vi "2016 Auto Drive Arm.vi"(0 "Left Side Speed":dbl, 2 "Right Side Speed":dbl, 3 "Arm Reference":T1, 5 "Arm Limits":T2, 6 "Left Side Reset":bool, 7 "Right Side Reset":bool, 8 "Left Upper Limit":dbl, 9 "Right Upper Limit":dbl, 10 "Left Lower Limit":dbl, 11 "Right Lower Limit":dbl) -> (14 "Encoder Status":T4, 16 "Encoder Status 2":T4, 19 "Arm Data":T3)   [LabVIEW 2015]
uses:
  <vilib>/Rock Robotics/WPI/Utilities/WPI_GetSetVariantRefNum.vi
  <vilib>/Rock Robotics/Network Tables/SD Write Numeric Array.vi
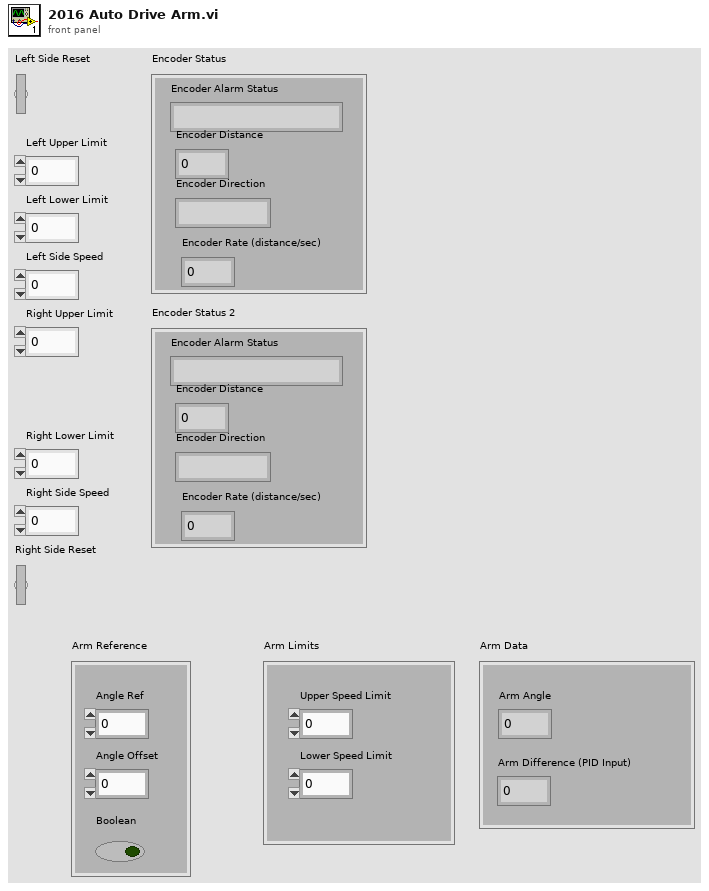
[diagram p1: front panel]
types:
  T1 = cluster{"Angle Ref":dbl, "Angle Offset":dbl, "Boolean":bool}
  T2 = cluster{"Upper Speed Limit":dbl, "Lower Speed Limit":dbl}
  T3 = cluster{"Arm Angle":dbl, "Arm Difference (PID Input)":dbl}
  T4 = cluster{"Encoder Alarm Status":string, "Encoder Distance":dbl, "Encoder Direction":string, "Encoder Rate (distance/sec)":dbl}
  T5 = typedef "WPI_PotentiometerDevRef.ctl" = cluster{"DevStatus":errorcluster, "Analog Channel":T6, "Invert Output":bool}
  T6 = typedef "FPGA_AIChannel.ctl" = enum8{"AI 0", "AI 1", "AI 2", "AI 3", "AI MXP 0", "AI MXP 1", "AI MXP 2", "AI MXP 3", "Invalid"}
  T7 = cluster{"P Gain":dbl, "I Gain":dbl, "D Gain":dbl, "t":dbl}
  T8 = cluster{"Arm Angle":dbl, "Angle Difference (PID Ref)":dbl}
  T9 = cluster{dbl, "Output offset":dbl, "Left Side Reset":bool}
  T10 = cluster{dbl, "Output offset":dbl, "Right Side Reset":bool}
  T11 = cluster{"Right Up Limit":dbl, "Right Lwr Limit":dbl}
  T12 = cluster{"Left Up Limit":dbl, "Left Lwr Limit":dbl}
  T13 = typedef "WPI_RobotDriveDevRef.ctl" = cluster{"DevStatus":errorcluster, "Motors[]":T14[], "Square Inputs":bool, "Max Output":dbl}
  T14 = typedef "WPI_MotorControlDeviceRef.ctl" = cluster{"DeviceStatus":errorcluster, "Type":T15, "PWM":cluster{"PWM Channel":T16, "DeadBand":T17}, "CAN":cluster{"Device Number":u8, "Control Mode":T18, "Semaphore":T19, "Max Vout":dbl, "TalonSRX Control Mode":T20}, "Invert":bool}
  T15 = typedef "WPI_MotorControlType.ctl" = enum16{"PWM", "CAN", "CANTalonSRX"}
  T16 = typedef "FPGA_DIOPWMChannel.ctl" = enum8{"PWM 0", "PWM 1", "PWM 2", "PWM 3", "PWM 4", "PWM 5", "PWM 6", "PWM 7", "PWM 8", "PWM 9", "PWM MXP 0", "PWM MXP 1", "PWM MXP 2", "PWM MXP 3", "PWM MXP 4", "PWM MXP 5", "PWM MXP 6", "PWM MXP 7", "PWM MXP 8", "PWM MXP 9", "Invalid"}
  T17 = typedef "WPI_PWMDeadband.ctl" = cluster{"Name":string, "maxPositivePwm":i32, "minPositivePwm":i32, "centerPwm":i32, "maxNegativePwm":i32, "minNegativePwm":i32, "angularRange":u16}
  T18 = typedef "WPI_CANJaguar_ControlMode.ctl" = enum8{"Percent VBus", "Current", "Speed", "Position", "Voltage"}
  T19 = typedef "Semaphore RefNum" = refnum<k1>
  T20 = typedef "WPI_CANTalonSRX_APIControlMode.ctl" = enum8{"Percent VBus", "Speed", "Position", "Slave", "Unchanged / Invalid", "Voltage Compensation", "Current", "Motion Profile"}
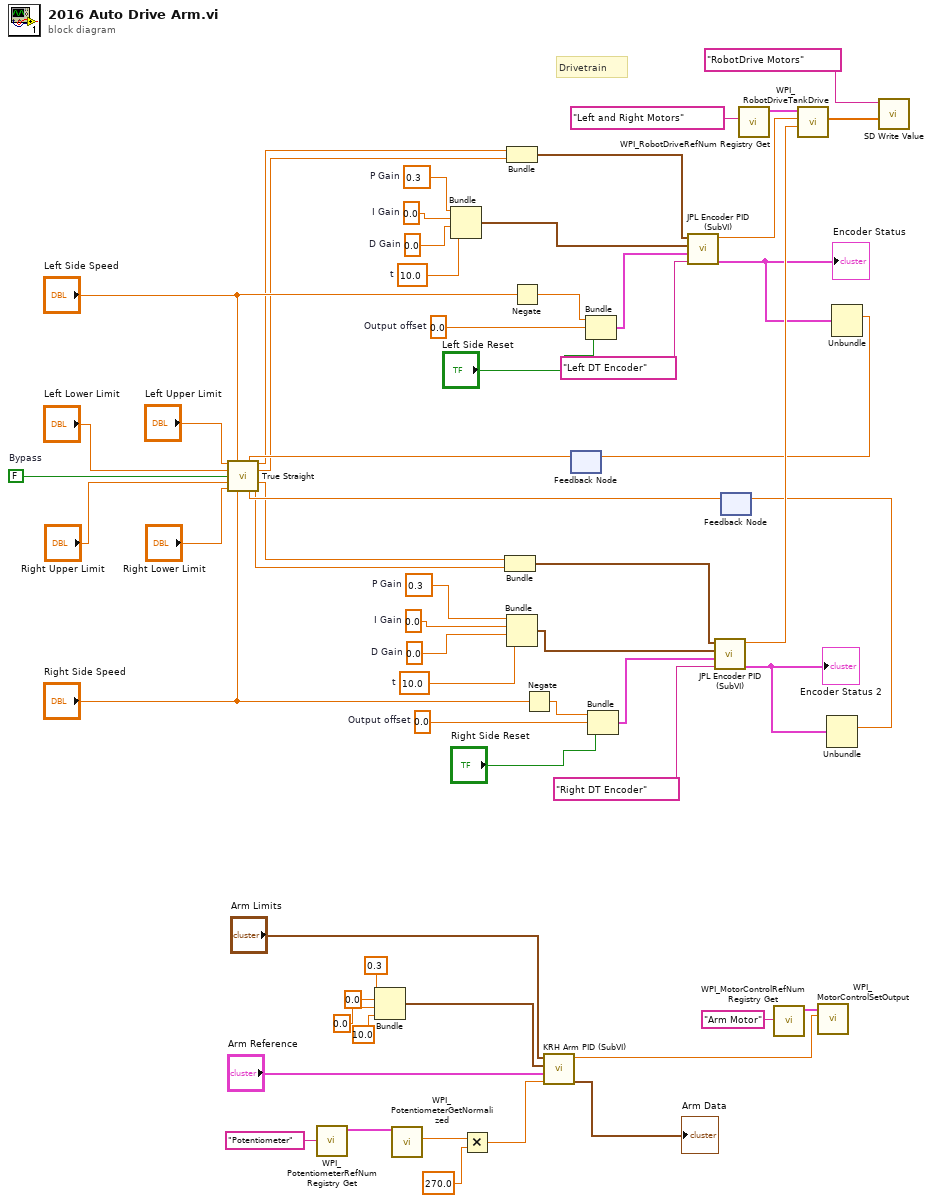
[diagram p0: block diagram]
diagram:
  w17 = FALSE  # Bypass
  w55 = 10.0  # t
  w54 = 0.0  # D Gain
  w53 = 0.0  # I Gain
  w52 = 0.3  # P Gain
  w51 = 0.0  # Output offset
  w46 = 10.0  # t
  w45 = 0.0  # D Gain
  w44 = 0.0  # I Gain
  w43 = 0.3  # P Gain
  w42 = 0.0  # Output offset
  # "Drivetrain"
  n1 = call <vilib>:"WPI_PotentiometerRefNum Registry Get.vi"("refnum name"="Potentiometer") -> ("PotDevRef"=w7:T5)  [unwired: 9 in, 1 out]
  n2 = Bundle(0.3, 0.0, 0.0, 10.0) -> (w16:cluster{dbl, dbl, dbl, dbl})  [unwired: 1 in]
  n3 = call <vilib>:"WPI_PotentiometerGetNormalized.vi"("PotDevRef"=w7) -> ("Normalized Value"=w8:dbl)  [unwired: 8 in, 2 out]
  n4 = Bundle("P Gain"=w43, "I Gain"=w44, "D Gain"=w45, "t"=w46) -> (w49:T7)  [unwired: 1 in]
  n5 = Multiply(x=w8, y=270.0) -> (x*y=w5:dbl)
  n6 = Bundle("P Gain"=w52, "I Gain"=w53, "D Gain"=w54, "t"=w55) -> (w58:T7)  [unwired: 1 in]
  n7 = Negate(x="Left Side Speed") -> (-x=w35:dbl)
  n8 = Negate(x="Right Side Speed") -> (-x=w34:dbl)
  n9 = call "KRH Arm PID (SubVI).vi"("Actual Angle"=w5, "Arm Control"="Arm Reference", "PID Settings"=w16, "PID Limits"="Arm Limits") -> ("Arm Status"=→"Arm Data":T8, "output"=w9:dbl)  [unwired: 2 in]
  n10 = feedback #1() -> (w27:dbl)  [unwired: 1 in]
  n11 = Bundle(w35, "Output offset"=w42, "Left Side Reset"="Left Side Reset") -> (w48:T9)  [unwired: 1 in]
  n12 = Bundle(w34, "Output offset"=w51, "Right Side Reset"="Right Side Reset") -> (w57:T10)  [unwired: 1 in]
  n13 = feedback #2() -> (w30:dbl)  [unwired: 1 in]
  n14 = call "True Straight.vi"("Left Upper Limit"="Left Upper Limit", "Left Speed"="Left Side Speed", "Left Encoder"=w27, "Left Lower Limit"="Left Lower Limit", "Bypass"=w17, "Right Upper Limit"="Right Upper Limit", "Right Lower Limit"="Right Lower Limit", "Right Speed"="Right Side Speed", "Right Encoder 2"=w30) -> ("Left Up Limit"=w21:dbl, "Left Lwr Limit"=w20:dbl, "Right Up Limit"=w19:dbl, "Right Lwr Limit"=w18:dbl)  [unwired: 3 in]
  n15 = Bundle("Right Up Limit"=w19, "Right Lwr Limit"=w18) -> (w59:T11)  [unwired: 1 in]
  n16 = Bundle("Left Up Limit"=w21, "Left Lwr Limit"=w20) -> (w50:T12)  [unwired: 1 in]
  n17 = call "JPL Encoder PID (SubVI).vi"("refnum name"="Left DT Encoder", "Encoder Config"=w48, "PID Settings"=w49, "PID Limits"=w50) -> ("Encoder Status"=w32:T4, "output"=w40:dbl)  [unwired: 2 in]
  "Encoder Status" <- w32
  n18 = call "JPL Encoder PID (SubVI).vi"("refnum name"="Right DT Encoder", "Encoder Config"=w57, "PID Settings"=w58, "PID Limits"=w59) -> ("Encoder Status"=w33:T4, "output"=w41:dbl)  [unwired: 2 in]
  "Encoder Status 2" <- w33
  n19 = call <vilib>:"WPI_RobotDriveRefNum Registry Get.vi"("refnum name"="Left and Right Motors") -> ("RobotDriveDevRef"=w37:T13)  [unwired: 1 in, 9 out]
  n20 = call <vilib>:"WPI_MotorControlRefNum Registry Get.vi"("refnum name"="Arm Motor") -> ("MotorControlDevRef"=w10:T14)  [unwired: 9 in, 1 out]
  n21 = call <vilib>:"WPI_RobotDriveTankDrive.vi"("Right axis value"=w41, "Left axis value"=w40, "RobotDriveDevRef"=w37) -> ("Motor Values"=w38:dbl[])  [unwired: 6 in, 2 out]
  n22 = call <vilib>:"WPI_MotorControlSetOutput.vi"("Output"=w9, "MotorControlDevRef"=w10) -> ()  [unwired: 7 in, 3 out]
  n23 = Unbundle(w33) -> ("Encoder Distance"=w31:dbl)  [unwired: 3 out]
  n24 = feedback-in #2(w31) -> ()
  n25 = Unbundle(w32) -> ("Encoder Distance"=w28:dbl)  [unwired: 3 out]
  n26 = feedback-in #1(w28) -> ()
  n27 = call-poly <vilib>:"SD Write Value.vi"("Numeric Array"=w38, "Name"="RobotDrive Motors") -> ()  [unwired: 8 in, 2 out]
